vi "AlliGator Get Series Analysis Type.vi"(11 "Menu Tag":string) -> (3 "Series Analysis Type":T1)   [LabVIEW 2021, in "AlliGator Scripts.lvlib"]
doc: "Decodes menu tag to determine whether an action is limited to the <B>Current ROI</B> or <B>All ROIs</B>."
uses:
  AlliGator Scripts.lvlib
  AlliGator Series Analysis Type.ctl
panel:
  # "see the AlliGator License on the block diagram (Ctrl+E or Window:Show Block Diagram)"
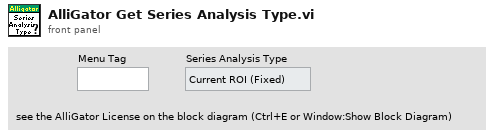
[diagram p1: front panel]
types:
  T1 = typedef "AlliGator Scripts.lvlib/AlliGator Series Analysis Type.ctl" = enum16{"Current ROI (Fixed)", "All ROIs (Fixed)", "Sequential ROIs"}
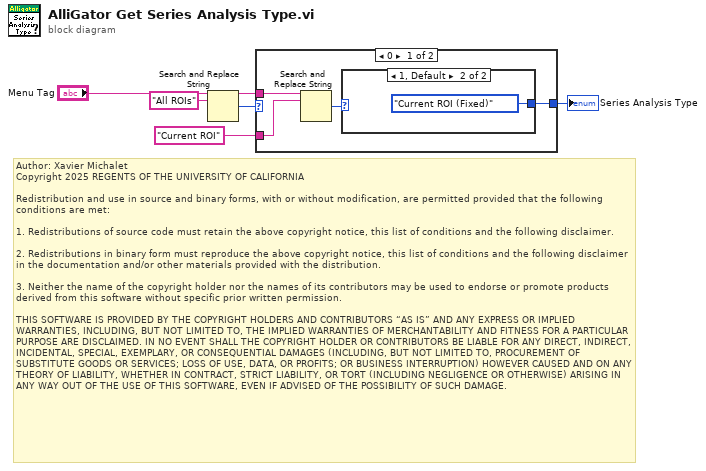
[diagram p0: block diagram]
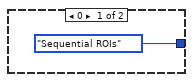
[diagram p2: hidden frame]
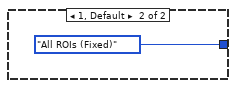
[diagram p3: hidden frame]
diagram:
  # "Author: Xavier Michalet\nCopyright 2025 REGENTS OF THE UNIVERSITY OF CALIFORNIA\n\nRedistribution and use in source and binary forms, with or without modification, are permitted provided that the following conditions are met:\n\n1. Redistributions of source code must retain the above copyright notice, this list of conditions and the following disclaimer.\n\n2. Redistributions in binary form must reproduce the above copyright notice, this list of conditions and the following disclaimer in the documentation and/or other materials provided with the distribution.\n\n3. Neither the name of the copyright holder nor the names of its contributors may be used to endorse or promote products derived from this software without specific prior written permission.\n\nTHIS SOFTWARE IS PROVIDED BY THE COPYRIGHT HOLDERS AND CONTRIBUTORS “AS IS” AND ANY EXPRESS OR IMPLIED WARRANTIES, INCLUDING, BUT NOT LIMITED TO, THE IMPLIED WARRANTIES OF MERCHANTABILITY AND FITNESS FOR A PARTICULAR PURPOSE ARE DISCLAIMED. IN NO EVENT SHALL THE COPYRIGHT HOLDER OR CONTRIBUTORS BE LIABLE FOR ANY DIRECT, INDIRECT, INCIDENTAL, SPECIAL, EXEMPLARY, OR CONSEQUENTIAL DAMAGES (INCLUDING, BUT NOT LIMITED TO, PROCUREMENT OF SUBSTITUTE GOODS OR SERVICES; LOSS OF USE, DATA, OR PROFITS; OR BUSINESS INTERRUPTION) HOWEVER CAUSED AND ON ANY THEORY OF LIABILITY, WHETHER IN CONTRACT, STRICT LIABILITY, OR TORT (INCLUDING NEGLIGENCE OR OTHERWISE) ARISING IN ANY WAY OUT OF THE USE OF THIS SOFTWARE, EVEN IF ADVISED OF THE POSSIBILITY OF SUCH DAMAGE."
  n1 = Search and Replace String(input string="Menu Tag", search string="All ROIs") -> (result string=w5:string, number of replacements=w3:i32)  [unwired: 6 in, 2 out]
  n2 = case shown="0" w3 {
    tunnel: [w7 AlliGator_Series_Analysis_Type."All ROIs (Fixed)"] -> w4
    tunnel: w5 -> [w10 _]
    tunnel: "Current ROI" ("search string") -> [w9 _]
    frame 0 {
      n3 = Search and Replace String(input string=w10, search string=w9) -> (number of replacements=w8:i32)  [unwired: 6 in, 3 out]
      n4 = case shown="1, Default" w8 {
        tunnel: [AlliGator_Series_Analysis_Type."Sequential ROIs" AlliGator_Series_Analysis_Type."Current ROI (Fixed)"] -> w7
        frame 0 {
        }
        frame 1, Default {
        }
      }
    }
    frame 1, Default {
    }
  }
  "Series Analysis Type" <- w4
